vi "mupSetLocale.vi"(8 "error in (no error)":errorcluster, 10 "Use system decimal point (T)":bool=TRUE, 11 "hParser in":u64) -> (0 "error out":errorcluster, 3 "hParser out":u64)   [LabVIEW 2015, in "mupLib.lvlib"]
doc: "Set to true to use system's decimal point.\n\nIf the system's decimal point is a comma, the argument separator will be changed to a semi-colon.\n\nThe default decimal point is a period. The default argument separator is a comma."
uses:
  mupLib.lvlib
panel:
  # "Set to true to use system's decimal point.\n\nIf the system's decimal point is a comma, the argument separator will be changed to a semi-colon.\n\nThe default decimal point is a period. The default argument separator is a comma."
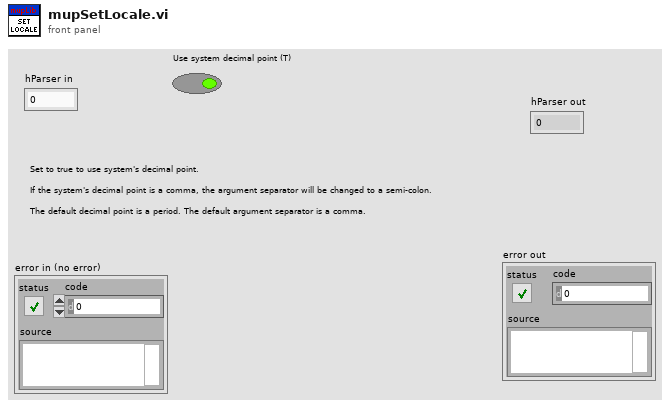
[diagram p1: front panel]
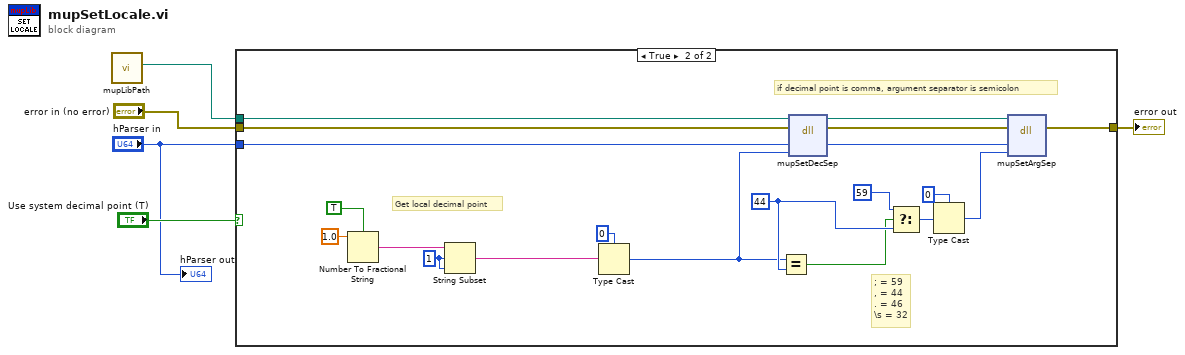
[diagram p0: block diagram]
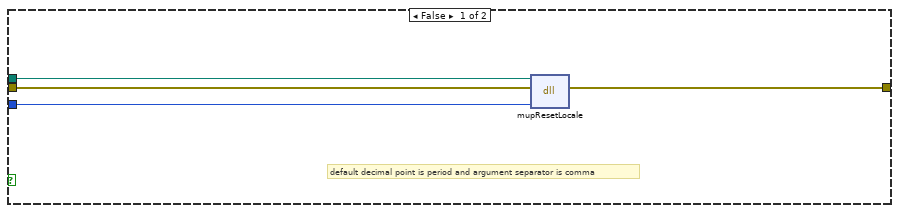
[diagram p2: hidden frame]
diagram:
  n1 = call "mupLibPath.vi"() -> ("libmuparser path"=w1:path)  [unwired: 11 in]
  n2 = case shown="True" "Use system decimal point (T)" {
    tunnel: [w7 w28] -> w5
    tunnel: "error in (no error)" -> [w9 w18]
    tunnel: "hParser in" -> [w8 w19]
    tunnel: w1 -> [w6 w11]
    frame False {
      # "default decimal point is period and argument separator is comma"
      n3 = dll-call lib="usr/lib/x86_64-linux-gnu/libmuparser.so.2" fn="mupResetLocale"(path in=w6, error in=w9, "hParser"=w8) -> (error out=w7:errorcluster)  [unwired: 3 in, 1 out]
    }
    frame True {
      w13 = 1 ("offset (0)")
      w22 = u8 44 ("y")
      # "if decimal point is comma, argument separator is semicolon"
      # "Get local decimal point"
      # "; = 59\n, = 44\n. = 46\n\\s = 32"
      n4 = Number To Fractional String(use system decimal point (T)=TRUE, number=1.0) -> (F-format string=w14:string)  [unwired: 2 in]
      n5 = String Subset(string=w14, offset (0)=w13, length (rest)=w13) -> (substring=w12:string)
      n6 = Type Cast(type=u8 0, x=w12) -> (*(type *) &x=w20:u8)
      n7 = Equal?(x=w20, y=w22) -> (x = y?=w17:bool)
      n8 = dll-call lib="usr/lib/x86_64-linux-gnu/libmuparser.so.2" fn="mupSetDecSep"(path in=w11, error in=w18, "hParser"=w19, "szChar"=w20) -> (path out=w10:path, error out=w29:errorcluster, "hParser"=w24:u64)  [unwired: 3 in]
      n9 = Select(t=u8 59 ("y"), s=w17, f=w22) -> (s? t:f=w26:u8)
      n10 = Type Cast(type=u8 0, x=w26) -> (*(type *) &x=w25:u8)
      n11 = dll-call lib="usr/lib/x86_64-linux-gnu/libmuparser.so.2" fn="mupSetArgSep"(path in=w10, error in=w29, "hParser"=w24, "szChar"=w25) -> (error out=w28:errorcluster)  [unwired: 4 in, 1 out]
    }
  }
  "error out" <- w5
  "hParser out" <- "hParser in"
